vi "rs3 delete frame queue2.vi"(8 "error in (no error)":errorcluster, 11 "queue":u64) -> (0 "error out":errorcluster)   [LabVIEW 2023]
doc: "Delete the queue, when done with it."
panel:
  # "RS Delete Frame Queue"
  # "(C) Intel Corp. 2017,  AGJ"
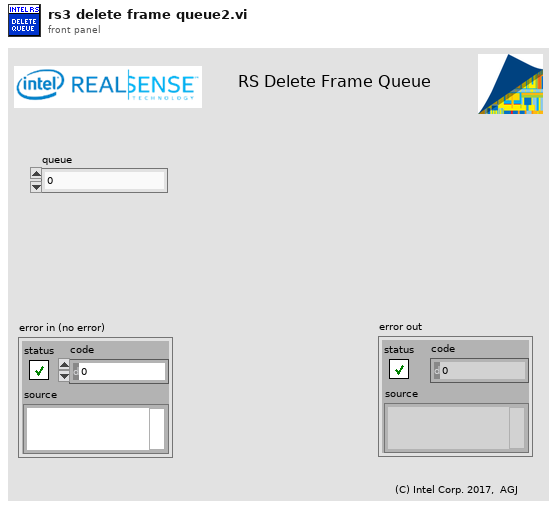
[diagram p1: front panel]
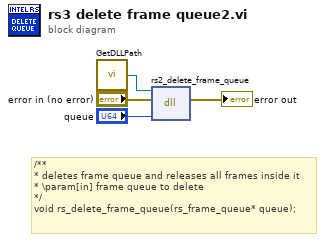
[diagram p0: block diagram]
diagram:
  # "/**\n* deletes frame queue and releases all frames inside it\n* \\param[in] frame queue to delete\n*/\nvoid rs_delete_frame_queue(rs_frame_queue* queue);"
  n1 = call "GetDLLPath.vi"() -> ("DLL Path"=w1:path)
  n2 = dll-call lib="C:/STEAMSyndicate/RealSenseWrappers/VI Wrappers (add ons) Public/RealSense/realsense2.dll" fn="rs2_delete_frame_queue"(path in=w1, error in="error in (no error)", "queue"="queue") -> (error out=→"error out":errorcluster)  [unwired: 3 in, 1 out]
